vi "ArmHome.vi"(0 "arm rotate motor devref":T2={"DeviceStatus"={"status"=FALSE, "code"=0, "source"=""}, "Type"=enum."PWM", "PWM"={"PWM Channel"=enum."Invalid", "DeadBand"={"Name"="", "maxPositivePwm"=0, "minPositivePwm"=0, "centerPwm"=0, "maxNegativePwm"=0, "minNegativePwm"=0, "angularRange"=0}}, "CAN"={"Device Number"=0, "SetOutput VI Ref"=variant(enum8{"Percent VBus", "Current", "Speed", "Position", "Voltage"} enum."Percent VBus"), "GetOutput VI Ref"=variant(refnum<k1> refnum), "Enable VI Ref"=variant(dbl 12.0), "Disable VI Ref"=variant(enum8{"Percent VBus", "Speed", "Position", "Slave", "Unchanged / Invalid", "Voltage Compensation", "Current", "Motion Profile"} enum."Percent VBus"), "Data"=variant}, "Invert"=FALSE, "DIO PWM"={"PWM \"Enable\" Channel"=enum."Invalid", "DIOChannel"=enum."Invalid", "PWM Rate"=0.0}}, 1 "RobotConfig":T7={"Motors"={"DriveLeftPrimary"={"CAN Address"=1, "Invert"=FALSE, "InvertSensor"=FALSE, "Unit Conversion Factor"=0.0, "Brake Mode"=enum."Override to Brake", "Reverse Limt Switch Mode"=enum."Normally Closed", "Forward Limt Swith Mode"=enum."Normally Closed", "PWM Channel"=enum."Invalid", "Motor Controller Type"=enum."Talon SRX"}, "DriveLeftSecondary1"={"CAN Address"=2, "Invert"=FALSE, "InvertSensor"=FALSE, "Unit Conversion Factor"=0.0, "Brake Mode"=enum."Override to Brake", "Reverse Limt Switch Mode"=enum."Normally Closed", "Forward Limt Swith Mode"=enum."Normally Closed", "PWM Channel"=enum."Invalid", "Motor Controller Type"=enum."Talon SRX"}, "DriveRightPrimary"={"CAN Address"=3, "Invert"=FALSE, "InvertSensor"=FALSE, "Unit Conversion Factor"=0.0, "Brake Mode"=enum."Override to Brake", "Reverse Limt Switch Mode"=enum."Normally Closed", "Forward Limt Swith Mode"=enum."Normally Closed", "PWM Channel"=enum."Invalid", "Motor Controller Type"=enum."Talon SRX"}, "DriveRightSecondary1"={"CAN Address"=4, "Invert"=FALSE, "InvertSensor"=FALSE, "Unit Conversion Factor"=0.0, "Brake Mode"=enum."Override to Brake", "Reverse Limt Switch Mode"=enum."Normally Closed", "Forward Limt Swith Mode"=enum."Normally Closed", "PWM Channel"=enum."Invalid", "Motor Controller Type"=enum."Talon SRX"}, "RightIntake"={"CAN Address"=8, "Invert"=FALSE, "InvertSensor"=FALSE, "Unit Conversion Factor"=0.0, "Brake Mode"=enum."Override to Brake", "Reverse Limt Switch Mode"=enum."Normally Closed", "Forward Limt Swith Mode"=enum."Normally Closed", "PWM Channel"=enum."Invalid", "Motor Controller Type"=enum."Talon SRX"}, "LeftIntake"={"CAN Address"=7, "Invert"=FALSE, "InvertSensor"=FALSE, "Unit Conversion Factor"=0.0, "Brake Mode"=enum."Override to Brake", "Reverse Limt Switch Mode"=enum."Normally Closed", "Forward Limt Swith Mode"=enum."Normally Closed", "PWM Channel"=enum."Invalid", "Motor Controller Type"=enum."Talon SRX"}, "ArmPivot"={"CAN Address"=5, "Invert"=FALSE, "InvertSensor"=FALSE, "Unit Conversion Factor"=0.0, "Brake Mode"=enum."Override to Brake", "Reverse Limt Switch Mode"=enum."Normally Closed", "Forward Limt Swith Mode"=enum."Normally Closed", "PWM Channel"=enum."Invalid", "Motor Controller Type"=enum."Talon SRX"}, "ArmExtend"={"CAN Address"=6, "Invert"=FALSE, "InvertSensor"=FALSE, "Unit Conversion Factor"=0.0, "Brake Mode"=enum."Override to Brake", "Reverse Limt Switch Mode"=enum."Normally Closed", "Forward Limt Swith Mode"=enum."Normally Closed", "PWM Channel"=enum."Invalid", "Motor Controller Type"=enum."Talon SRX"}, "ArmPivot2"={"CAN Address"=9, "Invert"=FALSE, "InvertSensor"=FALSE, "Unit Conversion Factor"=0.0, "Brake Mode"=enum."Override to Brake", "Reverse Limt Switch Mode"=enum."Normally Closed", "Forward Limt Swith Mode"=enum."Normally Closed", "PWM Channel"=enum."Invalid", "Motor Controller Type"=enum."Talon SRX"}, "Climber"={"CAN Address"=10, "Invert"=FALSE, "InvertSensor"=FALSE, "Unit Conversion Factor"=0.0, "Brake Mode"=enum."Override to Brake", "Reverse Limt Switch Mode"=enum."Disabled", "Forward Limt Swith Mode"=enum."Disabled", "PWM Channel"=enum."Invalid", "Motor Controller Type"=enum."Talon SRX"}, "Selfie Stick"={"CAN Address"=11, "Invert"=FALSE, "InvertSensor"=FALSE, "Unit Conversion Factor"=0.0, "Brake Mode"=enum."Override to Brake", "Reverse Limt Switch Mode"=enum."Disabled", "Forward Limt Swith Mode"=enum."Disabled", "PWM Channel"=enum."Invalid", "Motor Controller Type"=enum."Talon SRX"}}, "Sensors"={"IMU"={"Yaw Axis"=enum."Z", "SPI Bus"=enum."SPI MXP", "AHRS Algorithm"=enum."Complementary", "Calibration Time (s)"=3.0, "Calibrate On Open"=TRUE}, "LimitSwitch1"={"DIOChannel"=enum."DIO 0", "Active Low"=FALSE}, "LimitSwitch2"={"DIOChannel"=enum."DIO 1", "Active Low"=FALSE}, "BeamBreak"={"DIOChannel"=enum."DIO 2", "Active Low"=FALSE}, "JeVois"={"Baud Rate"=9600, "Parity"=0, "Data Bits"=8, "Stop Bits"=10, "Termination Char (0xA = '\\n' = LF)"=10, "Enable Termination Char? (T)"=TRUE, "Flow Control"=0, "Timeout Value (ms)"=5000, "Serial Port"=enum."Onboard RS-232"}}, "PID"={"ArmExtend"={"P"=0.0, "I"=0.0, "D"=0.0, "F"=0.0, "IZone"=0.0}, "ArmRotate"={"P"=0.0, "I"=0.0, "D"=0.0, "F"=0.0, "IZone"=0.0}, "Drive"={"P"=0.0, "I"=0.0, "D"=0.0, "F"=0.0, "IZone"=0.0}, "DriveGyro Kp ((in/sec)/deg)"=0.0, "CameraPole"={"P"=0.0, "I"=0.0, "D"=0.0, "F"=0.0, "IZone"=0.0}}, "Solenoids"={"ArmClaw"={"Forward Channel"=enum."Solenoid 0", "Invert"=FALSE, "Reverse Channel"=enum."Solenoid 0"}, "IntakeExtend"={"Forward Channel"=enum."Solenoid 1", "Invert"=FALSE, "Reverse Channel"=enum."Solenoid 0"}, "IntakeOpen"={"Forward Channel"=enum."Solenoid 2", "Invert"=FALSE, "Reverse Channel"=enum."Solenoid 0"}, " Shifter"={"Forward Channel"=enum."Solenoid 3", "Invert"=FALSE, "Reverse Channel"=enum."Solenoid 0"}}, "RobotDimensions "={"Length"=0.0, "Height"=0.0, "HeightOfBumpers"=0.0, "DistanceFromFrameEdgeToPyramid "=0.0, "HeightOfFrameToIntake"=0.0, "EdgeOfFrameToOrigin"=0.0}, "ArmHomePosition"={"Angle (rad)"=0.0, "Radius (in)"=0.0}, "SelfieStickParams"={"Home Height (in)"=0.0, "CruiseVelocity"=0, "MaxAccel"=0, "Low Height (in)"=0.0, "High Height (in)"=0.0, "Mid Height (in)"=0.0}, "Enable Compressor"=TRUE} {"Sensors"."JeVois"."Flow Control" items=["None", "XON/XOFF", "RTS/CTS", "XON/XOFF & RTS/CTS", "DTR/DSR", "XON/XOFF & DTR/DSR"]; "Sensors"."JeVois"."Termination Char (0xA = '\\n' = LF)" format="%.0x"; "Sensors"."JeVois"."Stop Bits" items=["1.0"=10, "1.5"=15, "2.0"=20]; "Sensors"."JeVois"."Parity" items=["None", "Odd", "Even", "Mark", "Space"]}, 5 "arm extend motor devref":T2={"DeviceStatus"={"status"=FALSE, "code"=0, "source"=""}, "Type"=enum."PWM", "PWM"={"PWM Channel"=enum."Invalid", "DeadBand"={"Name"="", "maxPositivePwm"=0, "minPositivePwm"=0, "centerPwm"=0, "maxNegativePwm"=0, "minNegativePwm"=0, "angularRange"=0}}, "CAN"={"Device Number"=0, "SetOutput VI Ref"=variant(enum8{"Percent VBus", "Current", "Speed", "Position", "Voltage"} enum."Percent VBus"), "GetOutput VI Ref"=variant(refnum<k1> refnum), "Enable VI Ref"=variant(dbl 12.0), "Disable VI Ref"=variant(enum8{"Percent VBus", "Speed", "Position", "Slave", "Unchanged / Invalid", "Voltage Compensation", "Current", "Motion Profile"} enum."Percent VBus"), "Data"=variant}, "Invert"=FALSE, "DIO PWM"={"PWM \"Enable\" Channel"=enum."Invalid", "DIOChannel"=enum."Invalid", "PWM Rate"=0.0}}, 11 "start":bool, 12 "stop":bool) -> (4 "arm rotate speed":dbl, 6 "arm extend speed":dbl, 8 "complete":bool, 10 "failed":bool, 15 "arm homing state":T1)   [LabVIEW 2018]
uses:
  TypeDefs/ConfigComponents/Config_Robot.ctl
  ArgosLib/Config/ConfigComponents/TypeDefs/Config_Motor.ctl
  <vilib>/Rock Robotics/WPI/ThirdParty/Phoenix-LabVIEW/Motor Controller/Controls/CTRE_Phoenix_MotorControl_NeutralMode.ctl
  <vilib>/Rock Robotics/WPI/ThirdParty/Phoenix-LabVIEW/Motor Controller/Controls/CTRE_Phoenix_MotorControl_LimitSwitchNormal.ctl
  <vilib>/Rock Robotics/SystemInterfaces/DIO/FPGA_DIOPWMChannel.ctl
  ArgosLib/Config/ConfigComponents/TypeDefs/Config_MotorCtrlType.ctl
  ArgosLib/Config/ConfigComponents/TypeDefs/Config_IMU.ctl
  <vilib>/Rock Robotics/SystemInterfaces/spilib/spi_bus.ctl
  ArgosLib/Config/ConfigComponents/TypeDefs/Config_DigitalIO.ctl
  <vilib>/Rock Robotics/SystemInterfaces/DIO/FPGA_DIOChannel.ctl
  ArgosLib/Config/ConfigComponents/TypeDefs/Config_SerialPort.ctl
  <vilib>/Rock Robotics/WPI/SerialPort/WPI_SerialPort.ctl
  ArgosLib/Config/ConfigComponents/TypeDefs/Config_PIDParams.ctl
  ArgosLib/Config/ConfigComponents/TypeDefs/Config_DoubleSolenoid.ctl
  <vilib>/Rock Robotics/WPI/Solenoid/WPI_SolenoidChannel.ctl
  TypeDefs/ConfigComponents/Config_Dimensions.ctl
  TypeDefs/ConfigComponents/Config_ArmHome.ctl
  TypeDefs/ConfigComponents/Config_SelfieStick.ctl
  <vilib>/Rock Robotics/WPI/MotorControl/WPI_MotorControlDeviceRef.ctl
  <vilib>/Rock Robotics/WPI/MotorControl/WPI_MotorControlType.ctl
  <vilib>/Rock Robotics/WPI/PWM/WPI_PWMDeadband.ctl
  TypeDefs/ArmHomingState.ctl
  <vilib>/Rock Robotics/WPI/ThirdParty/Phoenix-LabVIEW/Motor Controller/Get/CTRE_Phoenix_MotorController_GetSelectedSensorData.vi
  <vilib>/Rock Robotics/WPI/ThirdParty/Phoenix-LabVIEW/Motor Controller/Get/CTRE_Phoenix_MotorController_GetLimitSwitchStates.vi
  ArgosLib/ArgosLib.lvlib
panel:
  in  "Stall Time(ms)":u32=500
  in  "StallSpeed (ticks/100uS)":i32=10
  in  "arm rotate homing speed":dbl=-0.2
  in  "arm extend homing speed":dbl=-0.2
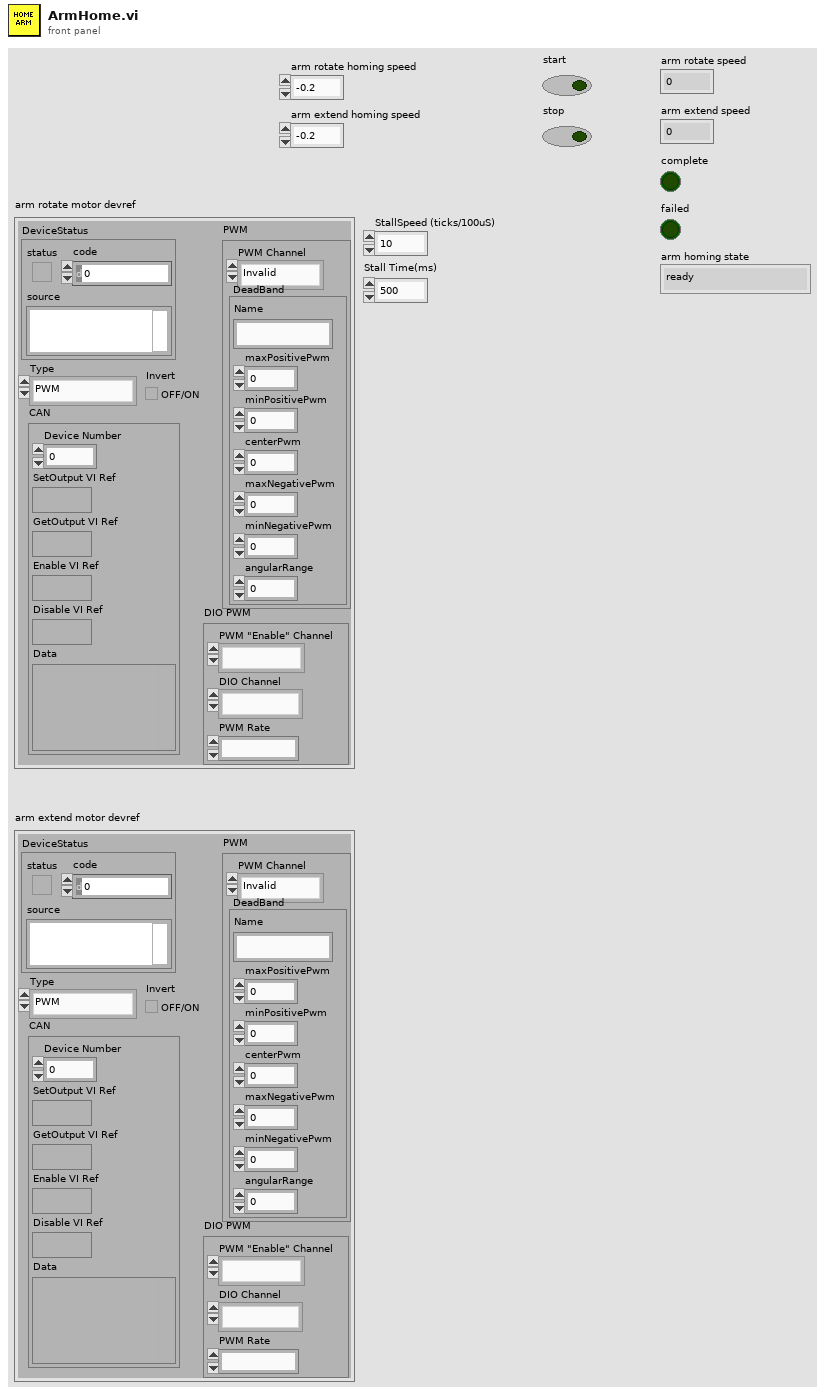
[diagram p1: front panel]
types:
  T1 = typedef "ArmHomingState.ctl" = enum16{"ready", "go to home", "homing complete ", "homing failed"}
  T2 = typedef "WPI_MotorControlDeviceRef.ctl" = cluster{"DeviceStatus":errorcluster, "Type":T3, "PWM":cluster{"PWM Channel":T4, "DeadBand":T5}, "CAN":cluster{"Device Number":u8, "SetOutput VI Ref":variant, "GetOutput VI Ref":variant, "Enable VI Ref":variant, "Disable VI Ref":variant, "Data":variant}, "Invert":bool, "DIO PWM":cluster{"PWM \"Enable\" Channel":T4, "DIOChannel":T6, "PWM Rate":dbl}}
  T3 = typedef "WPI_MotorControlType.ctl" = enum16{"PWM", "CAN", "DIO PWM"}
  T4 = typedef "FPGA_DIOPWMChannel.ctl" = enum8{"PWM 0", "PWM 1", "PWM 2", "PWM 3", "PWM 4", "PWM 5", "PWM 6", "PWM 7", "PWM 8", "PWM 9", "PWM MXP 0", "PWM MXP 1", "PWM MXP 2", "PWM MXP 3", "PWM MXP 4", "PWM MXP 5", "PWM MXP 6", "PWM MXP 7", "PWM MXP 8", "PWM MXP 9", "Invalid"}
  T5 = typedef "WPI_PWMDeadband.ctl" = cluster{"Name":string, "maxPositivePwm":i32, "minPositivePwm":i32, "centerPwm":i32, "maxNegativePwm":i32, "minNegativePwm":i32, "angularRange":u16}
  T6 = typedef "FPGA_DIOChannel.ctl" = enum8{"DIO 0", "DIO 1", "DIO 2", "DIO 3", "DIO 4", "DIO 5", "DIO 6", "DIO 7", "DIO 8", "DIO 9", "DIO MXP 0", "DIO MXP 1", "DIO MXP 2", "DIO MXP 3", "DIO MXP 4", "DIO MXP 5", "DIO MXP 6", "DIO MXP 7", "DIO MXP 8", "DIO MXP 9", "DIO MXP 10", "DIO MXP 11", "DIO MXP 12", "DIO MXP 13", "DIO MXP 14", "DIO MXP 15", "SPI Port CS1", "SPI Port CS2", "SPI Port CS3", "SPI Port MISO", "SPI Port MOSI", "Invalid"}
  T7 = typedef "Config_Robot.ctl" = cluster{"Motors":cluster{"DriveLeftPrimary":T8, "DriveLeftSecondary1":T8, "DriveRightPrimary":T8, "DriveRightSecondary1":T8, "RightIntake":T8, "LeftIntake":T8, "ArmPivot":T8, "ArmExtend":T8, "ArmPivot2":T8, "Climber":T8, "Selfie Stick":T8}, "Sensors":cluster{"IMU":T12, "LimitSwitch1":T14, "LimitSwitch2":T14, "BeamBreak":T14, "JeVois":T15}, "PID":cluster{"ArmExtend":T17, "ArmRotate":T17, "Drive":T17, "DriveGyro Kp ((in/sec)/deg)":dbl, "CameraPole":T17}, "Solenoids":cluster{"ArmClaw":T18, "IntakeExtend":T18, "IntakeOpen":T18, " Shifter":T18}, "RobotDimensions ":T20, "ArmHomePosition":T21, "SelfieStickParams":T22, "Enable Compressor":bool}
  T8 = typedef "ArgosLib.lvlib/Config_Motor.ctl" = cluster{"CAN Address":u8, "Invert":bool, "InvertSensor":bool, "Unit Conversion Factor":dbl, "Brake Mode":T9, "Reverse Limt Switch Mode":T10, "Forward Limt Swith Mode":T10, "PWM Channel":T4, "Motor Controller Type":T11}
  T9 = typedef "CTRE_Phoenix_MotorControl_NeutralMode.ctl" = enum8{"EEPROMSetting", "Override to Coast", "Override to Brake"}
  T10 = typedef "CTRE_Phoenix_MotorControl_LimitSwitchNormal.ctl" = enum16{"Normally Open", "Normally Closed", "Disabled"}
  T11 = typedef "ArgosLib.lvlib/Config_MotorCtrlType.ctl" = enum16{"Disabled", "Talon SRX", "Talon SR"}
  T12 = typedef "ArgosLib.lvlib/Config_IMU.ctl" = cluster{"Yaw Axis":enum16{"X", "Y", "Z"}, "SPI Bus":T13, "AHRS Algorithm":enum16{"Complementary", "Madgwick"}, "Calibration Time (s)":dbl, "Calibrate On Open":bool}
  T13 = typedef "spi_bus.ctl" = enum16{"SPI On-Board, CS0", "SPI On-Board, CS1", "SPI On-Board, CS2", "SPI On-Board, CS3", "SPI MXP", "Invalid"}
  T14 = typedef "ArgosLib.lvlib/Config_DigitalIO.ctl" = cluster{"DIOChannel":T6, "Active Low":bool}
  T15 = typedef "ArgosLib.lvlib/Config_SerialPort.ctl" = cluster{"Baud Rate":u32, "Parity":u16, "Data Bits":u16, "Stop Bits":u16, "Termination Char (0xA = '\\n' = LF)":u8, "Enable Termination Char? (T)":bool, "Flow Control":u16, "Timeout Value (ms)":u32, "Serial Port":T16}
  T16 = typedef "WPI_SerialPort.ctl" = enum16{"Onboard RS-232", "MXP TTL", "USB 1", "USB 2"}
  T17 = typedef "ArgosLib.lvlib/Config_PIDParams.ctl" = cluster{"P":dbl, "I":dbl, "D":dbl, "F":dbl, "IZone":dbl}
  T18 = typedef "ArgosLib.lvlib/Config_DoubleSolenoid.ctl" = cluster{"Forward Channel":T19, "Invert":bool, "Reverse Channel":T19}
  T19 = typedef "WPI_SolenoidChannel.ctl" = enum8{"Solenoid 0", "Solenoid 1", "Solenoid 2", "Solenoid 3", "Solenoid 4", "Solenoid 5", "Solenoid 6", "Solenoid 7", "Invalid"}
  T20 = typedef "Config_Dimensions.ctl" = cluster{"Length":dbl, "Height":dbl, "HeightOfBumpers":dbl, "DistanceFromFrameEdgeToPyramid ":dbl, "HeightOfFrameToIntake":dbl, "EdgeOfFrameToOrigin":dbl}
  T21 = typedef "Config_ArmHome.ctl" = cluster{"Angle (rad)":dbl, "Radius (in)":dbl}
  T22 = typedef "Config_SelfieStick.ctl" = cluster{"Home Height (in)":dbl, "CruiseVelocity":i32, "MaxAccel":i32, "Low Height (in)":dbl, "High Height (in)":dbl, "Mid Height (in)":dbl}
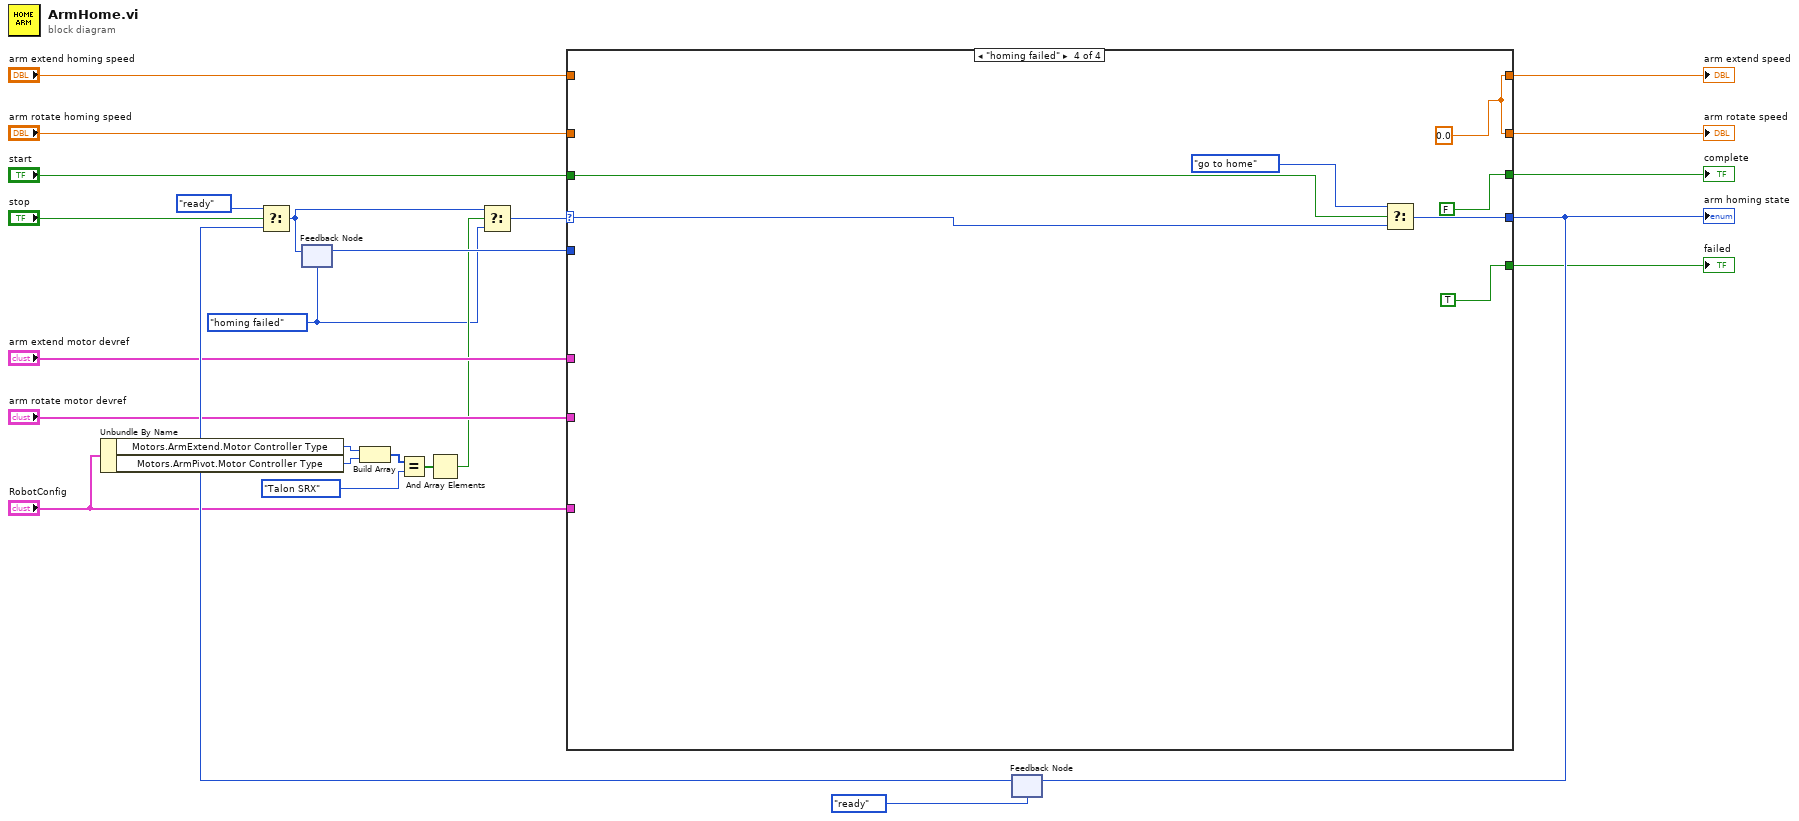
[diagram p0: block diagram]
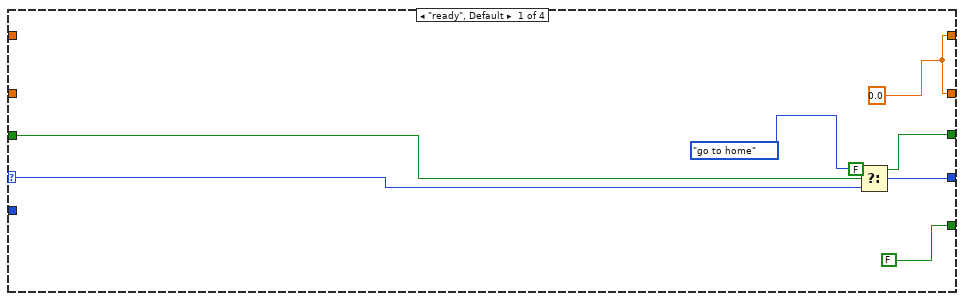
[diagram p2: hidden frame]
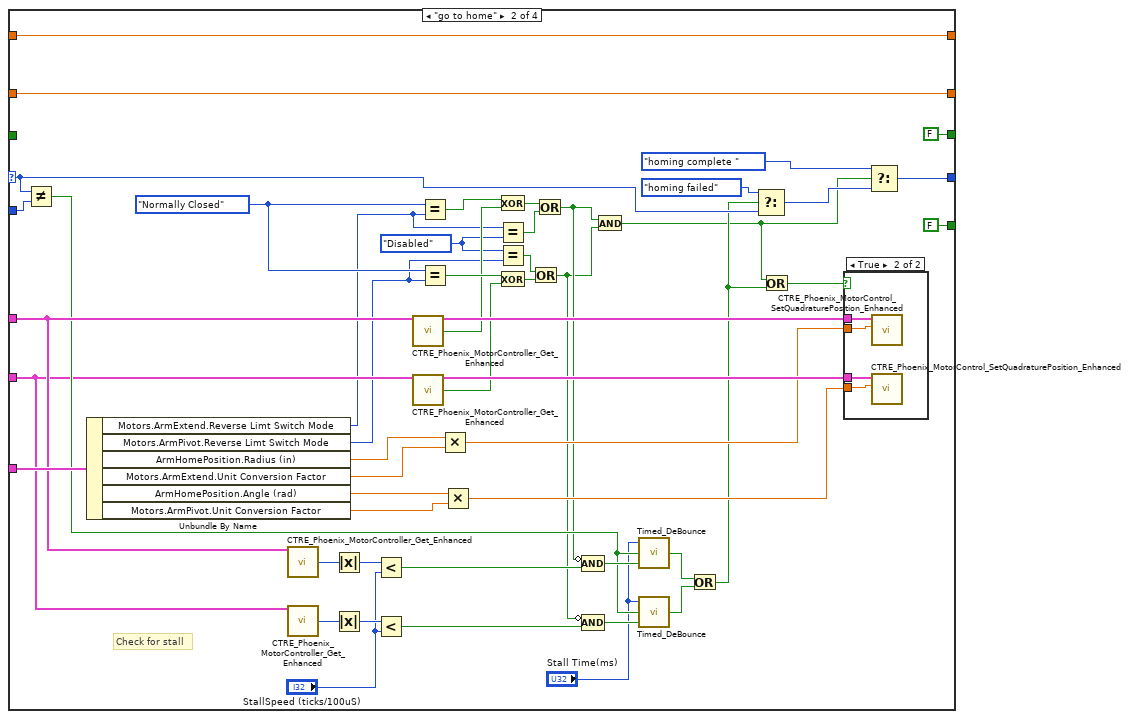
[diagram p3: hidden frame]
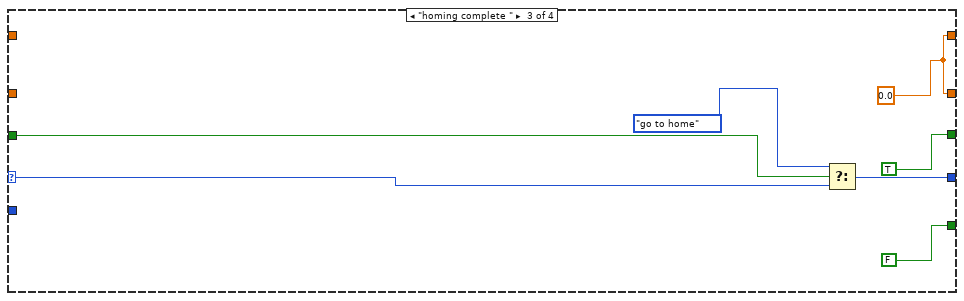
[diagram p5: hidden frame]
diagram:
  w1 = ArmHomingState."homing failed" ("arm homing state")
  n1 = Unbundle By Name("RobotConfig") -> ("Motors.ArmExtend.Motor Controller Type"=w8:T11, "Motors.ArmPivot.Motor Controller Type"=w7:T11)
  n2 = feedback #1(w1) -> (w11:T1)
  n3 = Build Array(w8, w7) -> (w6:T11[])
  n4 = Equal?(x=w6, y=Config_MotorCtrlType."Talon SRX" ("Motors.ArmPivot.Motor Controller Type")) -> (x = y?=w4:bool[])
  n5 = And Array Elements(Boolean array=w4) -> (logical AND=w2:bool)
  n6 = feedback #2(ArmHomingState."ready" ("arm homing state")) -> (w17:T1)
  n7 = Select(t=ArmHomingState."ready" ("arm homing state"), s="stop", f=w17) -> (s? t:f=w12:T1)
  n8 = feedback-in #1(w12) -> ()
  n9 = Select(t=w12, s=w2, f=w1) -> (s? t:f=w3:T1)
  n10 = case shown="\"homing failed\"" w3 {
    selector: w3 -> [w29 w49 w90 w97]
    tunnel: [w32 w83 w94 w101] -> w24
    tunnel: [w32 w82 w94 w101] -> w23
    tunnel: [FALSE FALSE TRUE FALSE] -> w22
    tunnel: [w30 w81 w92 w99] -> w21
    tunnel: "start" -> [w27 _ w91 w98]
    tunnel: "arm extend homing speed" -> [_ w83 _ _]
    tunnel: "arm rotate homing speed" -> [_ w82 _ _]
    tunnel: "arm extend motor devref" -> [_ w65 _ _]
    tunnel: "arm rotate motor devref" -> [_ w43 _ _]
    tunnel: "RobotConfig" -> [_ w77 _ _]
    tunnel: w11 -> [_ w55 _ _]
    tunnel: [FALSE FALSE FALSE TRUE] -> w10
    frame "ready", Default {
      w32 = 0.0
      n11 = Select(t=ArmHomingState."go to home", s=w27, f=w29) -> (s? t:f=w30:T1)
    }
    frame "go to home" {
      w33 = CTRE_Phoenix_MotorControl_LimitSwitchNormal."Disabled" ("y")
      w73 = CTRE_Phoenix_MotorControl_LimitSwitchNormal."Normally Closed" ("x")
      # "Check for stall"
      n12 = Not Equal?(x=w49, y=w55) -> (x != y?=w53:bool)
      n13 = Unbundle By Name(w77) -> ("Motors.ArmExtend.Reverse Limt Switch Mode"=w37:T10, "Motors.ArmPivot.Reverse Limt Switch Mode"=w34:T10, "ArmHomePosition.Radius (in)"=w68:dbl, "Motors.ArmExtend.Unit Conversion Factor"=w67:dbl, "ArmHomePosition.Angle (rad)"=w66:dbl, "Motors.ArmPivot.Unit Conversion Factor"=w76:dbl)
      n14 = call-poly <vilib>:"CTRE_Phoenix_MotorController_Get_Enhanced.vi"("PhoenixMotorControlDevRef"=w65) -> ("Velocity (Raw Sensor Units per 100 ms)"=w64:i32)  [unwired: 11 in, 3 out]
      n15 = call-poly <vilib>:"CTRE_Phoenix_MotorController_Get_Enhanced.vi"("PhoenixMotorControlDevRef"=w43) -> ("Velocity (Raw Sensor Units per 100 ms)"=w61:i32)  [unwired: 11 in, 3 out]
      n16 = Absolute Value(x=w64) -> (abs(x)=w63:i32)
      n17 = Absolute Value(x=w61) -> (abs(x)=w62:i32)
      n18 = Less?(x=w63, y="StallSpeed (ticks/100uS)") -> (x < y?=w58:bool)
      n19 = Less?(x=w62, y="StallSpeed (ticks/100uS)") -> (x < y?=w57:bool)
      n20 = call-poly <vilib>:"CTRE_Phoenix_MotorController_Get_Enhanced.vi"("PhoenixMotorControlDevRef"=w65) -> ("PhoenixMotorControlDevRef"=w79:T2, "Reverse Limit Closed?"=w69:bool)  [unwired: 11 in, 2 out]
      n21 = call-poly <vilib>:"CTRE_Phoenix_MotorController_Get_Enhanced.vi"("PhoenixMotorControlDevRef"=w43) -> ("PhoenixMotorControlDevRef"=w78:T2, "Reverse Limit Closed?"=w71:bool)  [unwired: 11 in, 2 out]
      n22 = Equal?(x=w73, y=w37) -> (x = y?=w70:bool)
      n23 = Equal?(x=w73, y=w34) -> (x = y?=w72:bool)
      n24 = Multiply(x=w68, y=w67) -> (x*y=w75:dbl)
      n25 = Multiply(x=w66, y=w76) -> (x*y=w74:dbl)
      n26 = Exclusive Or(1:w69, 2:w70) -> (0:w59:bool)
      n27 = Equal?(x=w37, y=w33) -> (x = y?=w35:bool)
      n28 = Equal?(x=w33, y=w34) -> (x = y?=w36:bool)
      n29 = Exclusive Or(1:w71, 2:w72) -> (0:w40:bool)
      n30 = Or(x=w36, y=w40) -> (x .or. y?=w38:bool)
      n31 = Or(x=w59, y=w35) -> (x .or. y?=w39:bool)
      n32 = Compound Arithmetic op=AND(invert w39, w58) -> (w56:bool)
      n33 = Compound Arithmetic op=AND(invert w38, w57) -> (w54:bool)
      n34 = And(x=w39, y=w38) -> (x .and. y?=w45:bool)
      n35 = call "Timed_DeBounce.vi"("Input"=w56, "Reset"=w53, "Hold Time(ms)"="Stall Time(ms)") -> ("Output"=w51:bool)
      n36 = call "Timed_DeBounce.vi"("Input"=w54, "Reset"=w53, "Hold Time(ms)"="Stall Time(ms)") -> ("Output"=w50:bool)
      n37 = Or(x=w51, y=w50) -> (x .or. y?=w46:bool)
      n38 = Select(t=ArmHomingState."homing failed", s=w46, f=w49) -> (s? t:f=w48:T1)
      n39 = Or(x=w45, y=w46) -> (x .or. y?=w44:bool)
      n40 = case shown="True" w44 {
        tunnel: w79 -> [_ w87]
        tunnel: w78 -> [_ w86]
        tunnel: w75 -> [_ w85]
        tunnel: w74 -> [_ w84]
        frame False {
        }
        frame True {
          n41 = call <vilib>:"CTRE_Phoenix_MotorControl_SetQuadraturePosition_Enhanced.vi"("New Position"=w85, "PhoenixMotorControlDevRef"=w87) -> ()  [unwired: 8 in, 2 out]
          n42 = call <vilib>:"CTRE_Phoenix_MotorControl_SetQuadraturePosition_Enhanced.vi"("New Position"=w84, "PhoenixMotorControlDevRef"=w86) -> ()  [unwired: 8 in, 2 out]
        }
      }
      n43 = Select(t=ArmHomingState."homing complete ", s=w45, f=w48) -> (s? t:f=w81:T1)
    }
    frame "homing complete " {
      w94 = 0.0 ("arm extend homing speed")
      n44 = Select(t=ArmHomingState."go to home", s=w91, f=w90) -> (s? t:f=w92:T1)
    }
    frame "homing failed" {
      w101 = 0.0 ("arm extend homing speed")
      n45 = Select(t=ArmHomingState."go to home", s=w98, f=w97) -> (s? t:f=w99:T1)
    }
  }
  "complete" <- w22
  "arm rotate speed" <- w23
  "arm extend speed" <- w24
  "arm homing state" <- w21
  "failed" <- w10
  n46 = feedback-in #2(w21) -> ()
